vi "Read Single Digital Port.vi"() -> ()   [LabVIEW 2020]
uses:
  <instrlib>/BDAQ-6104/Examples/Read Single Digital Channel.vi
  <instrlib>/BDAQ-6104/BDAQ-6104.lvlib
panel:
  out "Pin State":bool
  in  "Pin Number":T1(ring)
  in  "VISA resource name":refnum<visa-resource-name>
  # "Reads the current state of the spcified \ndigital pin."
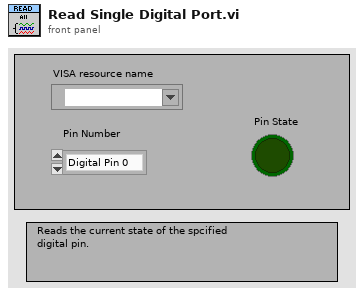
[diagram p1: front panel]
types:
  T1 = enum16{"Digital Pin 0", "Digital Pin 1", "Digital Pin 2", "Digital Pin 3"}
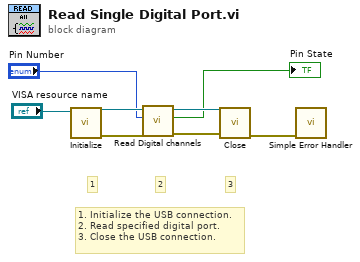
[diagram p0: block diagram]
diagram:
  # "1. Initialize the USB connection.\n2. Read specified digital port.\n3. Close the USB connection."
  # "3"
  # "2"
  # "1"
  n1 = call <instrlib>:"Initialize.vi"("VISA resource name"="VISA resource name") -> ("error out"=w6:errorcluster, "VISA resource name out"=w7:refnum<visa-resource-name>)  [unwired: 9 in]
  n2 = call-poly <instrlib>:"Read Digital channels.vi"("error in (no error)"=w6, "Pin Number"="Pin Number", "VISA resource name"=w7) -> ("error out"=w5:errorcluster, "Pin State"=→"Pin State":bool, "VISA resource name out"=w4:refnum<visa-resource-name>)  [unwired: 6 in]
  n3 = call <instrlib>:"Close.vi"("error in (no error)"=w5, "VISA resource name"=w4) -> ("error out"=w1:errorcluster)  [unwired: 9 in]
  n4 = call <vilib>:"Simple Error Handler.vi"("error in (no error)"=w1) -> ()  [unwired: 4 in, 5 out]
